vi "Get Scalar Data Variant.vi"(8 "error in (no error)":errorcluster, 9 "index":i32, 11 "Core Channels Configuration in":refnum<class "Core Channels Configuration.lvclass">) -> (0 "error out":errorcluster, 1 "data version":T1, 2 "data":variant, 3 "Core Channels Configuration out":refnum<class "Core Channels Configuration.lvclass">)   [LabVIEW 2017, in "DSF Core.lvlib" / "Core Channels Configuration.lvclass"]
uses:
  Core Channels Configuration.lvclass
  C:/Git/DSF/Core/Classes/Configuration/Configuration.lvclass
  Typedefs/DSF Version Info.ctl
  Configuration.lvclass
  DSF Core.lvlib
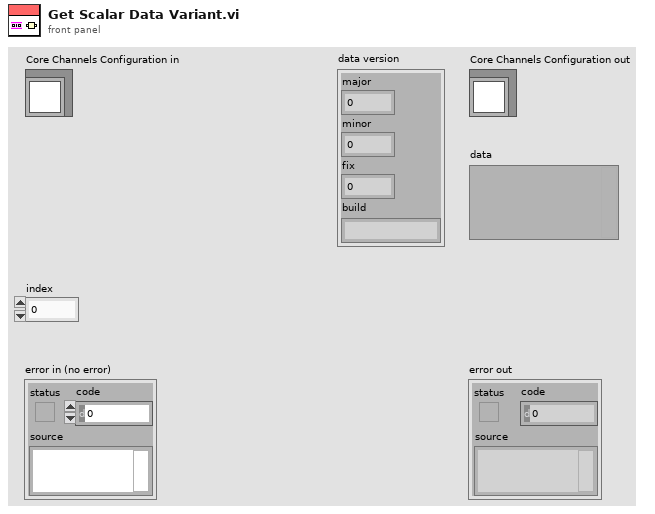
[diagram p1: front panel]
types:
  T1 = typedef "DSF Core.lvlib/DSF Version Info.ctl" = cluster{"major":u32, "minor":u32, "fix":u32, "build":string}
  T2 = typedef "DSF Core.lvlib/DSF Core Channel Configuration.ctl" = cluster{"name":string, "units":string, "engine data type":T3, "string data type":T3, "string offset":u64}
  T3 = typedef "DSF Core.lvlib/DSF Data Type.ctl" = enum8{"Bool", "SGL", "DBL", "I8", "I16", "I32", "I64", "U8", "U16", "U32", "U64"}
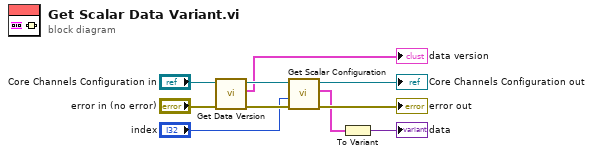
[diagram p0: block diagram]
diagram:
  n1 = call "Get Data Version.vi"("error in (no error)"="error in (no error)", "Configuration in"="Core Channels Configuration in") -> ("error out"=w5:errorcluster, "data version"=→"data version":T1, "Configuration out"=w8:refnum<class "Core Channels Configuration.lvclass">)  [unwired: 7 in]
  n2 = call "Get Scalar Configuration.vi"("error in (no error)"=w5, "index"="index", "Core Channel Configuration in"=w8) -> ("error out"=→"error out":errorcluster, "channel configuration"=w2:T2, "Core Channel Configuration out"=→"Core Channels Configuration out":refnum<class "Core Channels Configuration.lvclass">)  [unwired: 6 in]
  n3 = To Variant(anything=w2) -> (Variant=→"data":variant)
